vi "Cleanup.vi"(8 "error in (no error)":errorcluster, 11 "Node in":refnum<class "bt_Send_Queue.lvclass">) -> (0 "error out":errorcluster, 3 "Node out":refnum<class "bt_Send_Queue.lvclass">)   [LabVIEW 2021, in "BT.lvlib" / "bt_Send_Queue.lvclass"]
uses:
  bt_Send_Queue.lvclass
  With Values/Send/bt_Send_Synch_WithValues.lvclass
  bt_Send_Queue.lvclass/bt_Send_Queue.ctl
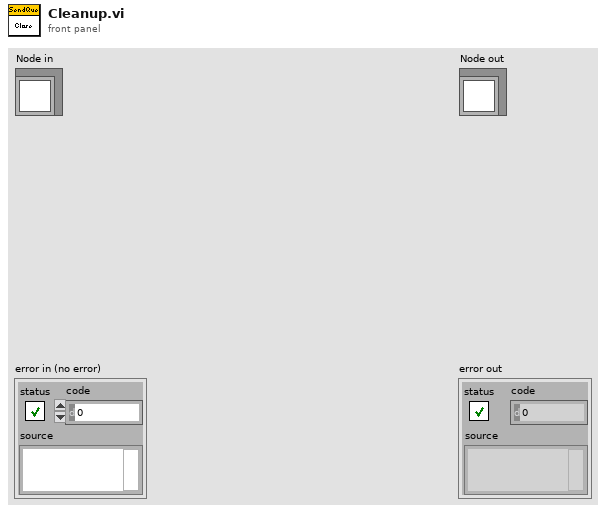
[diagram p1: front panel]
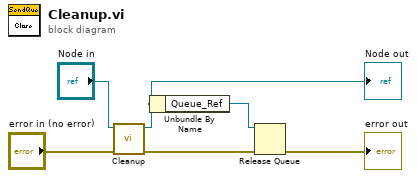
[diagram p0: block diagram]
diagram:
  n1 = call-parent "Cleanup.vi"("error in (no error)"="error in (no error)", "Node in"="Node in") -> ("error out"=w3:errorcluster, "Node out"=w4:refnum<class "bt_Send_Queue.lvclass">)  [unwired: 8 in]
  "Node out" <- w4
  n2 = Unbundle By Name(w4) -> ("Queue_Ref"=w2:refnum<queue>)
  n3 = Release Queue(queue=w2, error in (no error)=w3) -> (error out=→"error out":errorcluster)  [unwired: 1 in, 2 out]
